vi "Brew.vi"(8 "error in (no error)":errorcluster, 11 "CaffeineBeverage in":refnum<class "CaffeineBeverage.lvclass">) -> (0 "error out":errorcluster, 2 "ProcessMessage":string, 3 "CaffeineBeverage out":refnum<class "CaffeineBeverage.lvclass">)   [LabVIEW 2013, in "CaffeineBeverage.lvclass"]
uses:
  CaffeineBeverage.lvclass
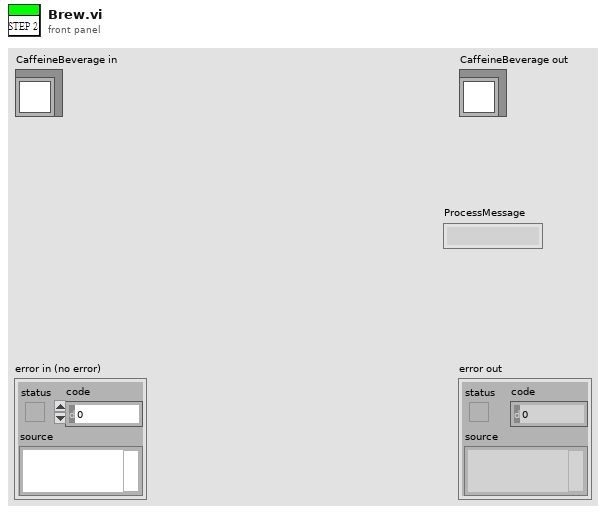
[diagram p1: front panel]
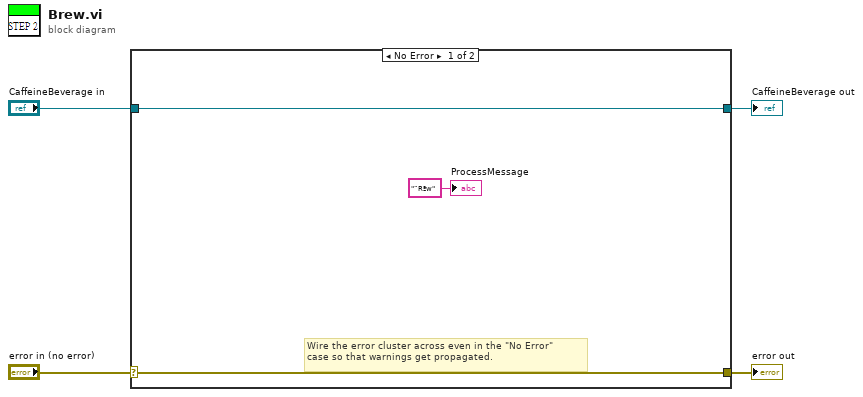
[diagram p0: block diagram]
diagram:
  n1 = case shown="No Error" "error in (no error)" {
    selector: "error in (no error)" -> [w6 w9]
    tunnel: [w6 w9] -> w3
    tunnel: [w7 w8] -> w1
    tunnel: "CaffeineBeverage in" -> [w7 w8]
    frame No Error {
      # "Wire the error cluster across even in the \"No Error\"\ncase so that warnings get propagated."
      "ProcessMessage" <- "¨Rªw" ("ProcessMessage")
    }
    frame Error {
    }
  }
  "error out" <- w3
  "CaffeineBeverage out" <- w1
